vi "Initialize CAN Message.vi"() -> (3 "Initial Payload":u8[](array[numeric]) format="%x")   [LabVIEW 2015, in "PAS.lvclass"]
uses:
  PAS.lvclass
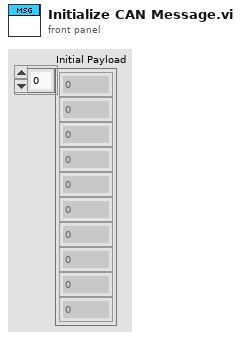
[diagram p1: front panel]
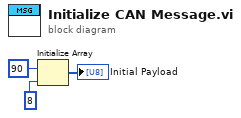
[diagram p0: block diagram]
diagram:
  n1 = Initialize Array(u8 90 ("Numeric"), 8 ("dimension size")) -> (→"Initial Payload":u8[])
